vi "Add Shapes.vi"(4 "event":enum16{"click", "mouse move", "enter", "leave"}(ring), 6 "Button":u16, 8 "error in (no error)":errorcluster, 9 "Coords":T1, 10 "XY Graph":refnum<vi>, 11 "input picture":picture) -> (0 "error out":errorcluster, 3 "output picture":picture)   [LabVIEW 2015]
uses:
  <vilib>/Utility/miscctls.llb/LVPoint32TypeDef.ctl
  <vilib>/Utility/cursorutil.llb/Set Cursor (Icon Pict).vi
panel:
  in  "Shape":T2(ring)
  in  "Postion":enum16{"freehand", "lock to plot"}(ring)
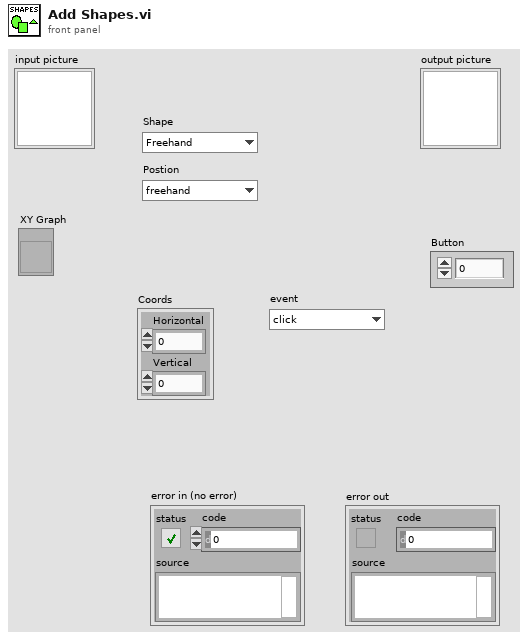
[diagram p1: front panel]
types:
  T1 = typedef "LVPoint32TypeDef.ctl" = cluster{"Horizontal":i32, "Vertical":i32}
  T2 = enum16{"Freehand", "Rectangle", "Oval", "Arc", "Line"}
  T3 = cluster{"left":i16, "top":i16, "right":i16, "bottom":i16}
  T4 = typedef "LVRectTypeDef.ctl" = cluster{"Left":i16, "Top":i16, "Right":i16, "Bottom":i16}
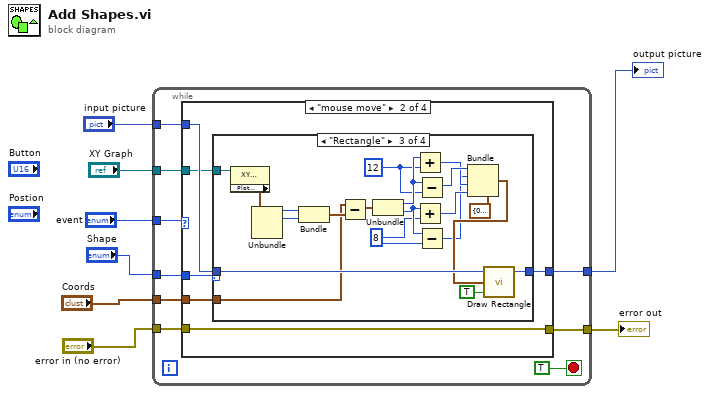
[diagram p0: block diagram]
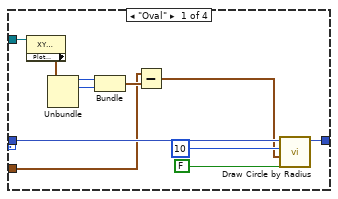
[diagram p3: hidden frame]
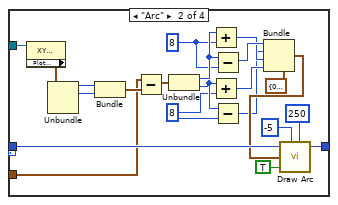
[diagram p4: hidden frame]
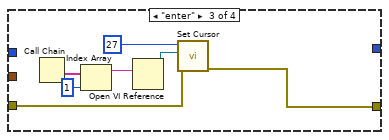
[diagram p6: hidden frame]
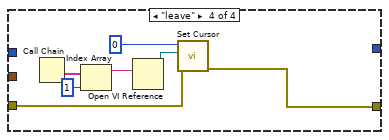
[diagram p7: hidden frame]
diagram:
  n1 = while {
    tunnel: "XY Graph" -> [w9]
    tunnel: "Coords" -> [w17]
    tunnel: "Shape" -> [w16]
    tunnel: "event" -> [w15]
    tunnel: "error in (no error)" -> [w14]
    tunnel: [w13] -> w3
    tunnel: [w11] -> w2
    tunnel: "input picture" -> [w10]
    stop <- TRUE stop-if-true
    n2 = case shown="\"mouse move\"" w15 {
      tunnel: w17 -> [_ w24 _ _]
      tunnel: w16 -> [_ w23 _ _]
      tunnel: w14 -> [w18 w22 w84 w91]
      tunnel: [w18 w22 w83 w90] -> w13
      tunnel: [_ w21 _ _] -> w11
      tunnel: w10 -> [_ w20 _ _]
      tunnel: w9 -> [_ w19 _ _]
      frame "click", Default {
      }
      frame "mouse move" {
        n3 = case shown="\"Rectangle\"" w23 {
          tunnel: w24 -> [w26 w50 w70 _]
          tunnel: [w34 w57 w77 w78] -> w21
          tunnel: w20 -> [w33 w56 w76 w78]
          tunnel: w19 -> [w28 w52 w72 _]
          frame "Oval" {
            n4 = property class="XYGraph"(reference=w28) -> ("Plot Bounds"=w27:T4)  [unwired: 1 in, 2 out]
            n5 = Unbundle(w27) -> ("Left"=w30:i16, "Top"=w31:i16)  [unwired: 2 out]
            n6 = Bundle("Left"=w30, "Top"=w31) -> (w29:cluster{"Left":i16, "Top":i16})  [unwired: 1 in]
            n7 = Subtract(x=w26, y=w29) -> (x-y=w25:T1)
            n8 = call <vilib>:"Draw Circle by Radius.vi"("fill?(F)"=FALSE, "pixel center"=w25, "radius"=i16 10, "picture"=w33) -> ("new picture"=w34:picture)  [unwired: 7 in]
          }
          frame "Arc" {
            w38 = 8 ("y")
            w42 = 8 ("y")
            n9 = property class="XYGraph"(reference=w52) -> ("Plot Bounds"=w51:T4)  [unwired: 1 in, 2 out]
            n10 = Unbundle(w51) -> ("Left"=w54:i16, "Top"=w55:i16)  [unwired: 2 out]
            n11 = Bundle("Left"=w54, "Top"=w55) -> (w53:cluster{"Left":i16, "Top":i16})  [unwired: 1 in]
            n12 = Subtract(x=w50, y=w53) -> (x-y=w46:T1)
            n13 = Unbundle(w46) -> ("Horizontal"=w43:i32, "Vertical"=w39:i32)
            n14 = Add(x=w43, y=w42) -> (x+y=w40:i32)
            n15 = Add(x=w39, y=w38) -> (x+y=w37:i32)
            n16 = Subtract(x=w43, y=w42) -> (x-y=w41:i32)
            n17 = Subtract(x=w39, y=w38) -> (x-y=w36:i32)
            n18 = Bundle(cluster=T3 {"left"=0, "top"=0, "right"=0, "bottom"=0} ("rect"), "left"=w41, "top"=w36, "right"=w40, "bottom"=w37) -> (w44:T3)
            n19 = call <vilib>:"Draw Arc.vi"("picture"=w56, "start angle[degrees]"=i16 -5 ("radius"), "rect"=w44, "fill?(F)"=TRUE, "arc size[degrees]"=i16 250) -> ("new picture"=w57:picture)  [unwired: 4 in]
          }
          frame "Rectangle" {
            w60 = 8 ("y")
            w64 = 12 ("y")
            n20 = property class="XYGraph"(reference=w72) -> ("Plot Bounds"=w71:T4)  [unwired: 1 in, 2 out]
            n21 = Unbundle(w71) -> ("Left"=w74:i16, "Top"=w75:i16)  [unwired: 2 out]
            n22 = Bundle("Left"=w74, "Top"=w75) -> (w73:cluster{"Left":i16, "Top":i16})  [unwired: 1 in]
            n23 = Subtract(x=w70, y=w73) -> (x-y=w68:T1)
            n24 = Unbundle(w68) -> ("Horizontal"=w65:i32, "Vertical"=w61:i32)
            n25 = Add(x=w65, y=w64) -> (x+y=w62:i32)
            n26 = Add(x=w61, y=w60) -> (x+y=w59:i32)
            n27 = Subtract(x=w65, y=w64) -> (x-y=w63:i32)
            n28 = Subtract(x=w61, y=w60) -> (x-y=w58:i32)
            n29 = Bundle(cluster=T3 {"left"=0, "top"=0, "right"=0, "bottom"=0} ("rect"), "left"=w63, "top"=w58, "right"=w62, "bottom"=w59) -> (w66:T3)
            n30 = call <vilib>:"Draw Rectangle.vi"("picture"=w76, "rect"=w66, "fill?(F)"=TRUE) -> ("new picture"=w77:picture)  [unwired: 6 in]
          }
          frame Default {
          }
        }
      }
      frame "enter" {
        n31 = Call Chain() -> (call chain=w82:string[])
        n32 = Index Array(array=w82, index=1) -> (element=w81:string)
        n33 = Open VI Reference(vi path=w81) -> (vi reference=w80:refnum<vi>)  [unwired: 5 in, 1 out]
        n34 = call-poly <vilib>:"Set Cursor.vi"("error in (no error)"=w84, "VI reference (current VI)"=w80, "icon"=u16 27) -> ("error out"=w83:errorcluster)  [unwired: 7 in, 1 out]
      }
      frame "leave" {
        n35 = Call Chain() -> (call chain=w89:string[])
        n36 = Index Array(array=w89, index=1) -> (element=w88:string)
        n37 = Open VI Reference(vi path=w88) -> (vi reference=w87:refnum<vi>)  [unwired: 5 in, 1 out]
        n38 = call-poly <vilib>:"Set Cursor.vi"("error in (no error)"=w91, "VI reference (current VI)"=w87, "icon"=u16 0) -> ("error out"=w90:errorcluster)  [unwired: 7 in, 1 out]
      }
    }
  }
  "error out" <- w3
  "output picture" <- w2
